vi "Set trigger.vi"(8 "error in (no error)":errorcluster, 11 "StageSPIM in":refnum<class "StageSPIM.lvclass">) -> (0 "error out":errorcluster, 3 "StageSPIM out":refnum<class "StageSPIM.lvclass">)   [LabVIEW 2012, in "StageSPIM.lvclass"]
uses:
  StageSPIM.lvclass
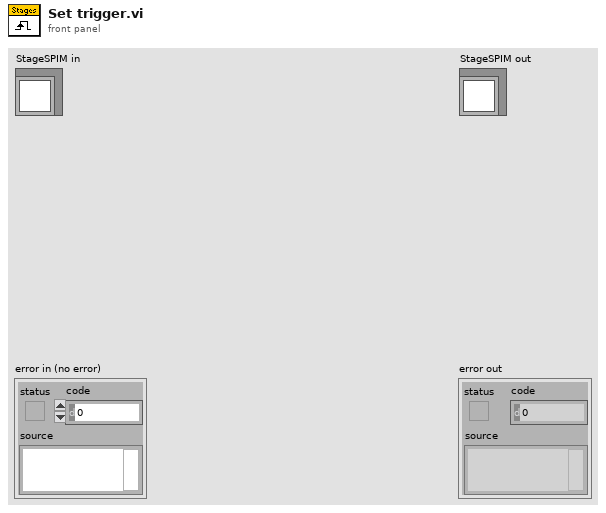
[diagram p1: front panel]
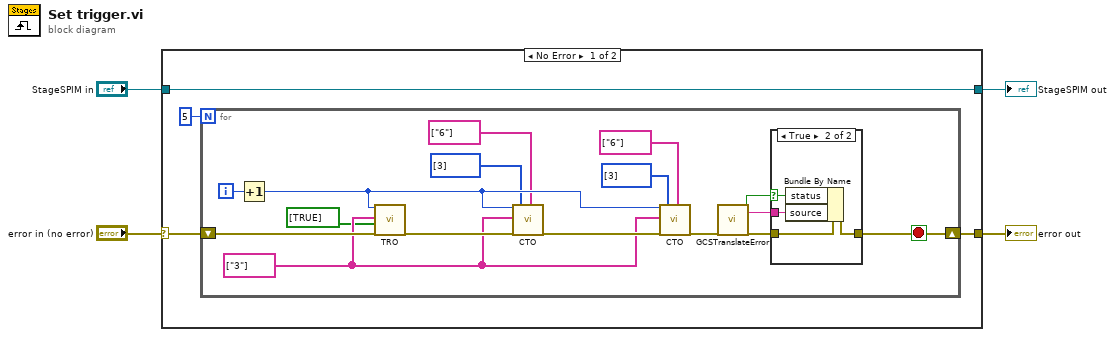
[diagram p0: block diagram]
diagram:
  n1 = case shown="No Error" "error in (no error)" {
    selector: "error in (no error)" -> [w6 w31]
    tunnel: [w5 w31] -> w3
    tunnel: [w8 w30] -> w1
    tunnel: "StageSPIM in" -> [w8 w30]
    frame No Error {
      n2 = for {
        N: 5 -> [_]
        shift-right: [w17] -> w5
        shift-left: w6 -> [w15]
        i -> [w24]
        stop <- w17 stop-if-true
        w13 = string[] ["3"] ("TriggerOut to set")
        n3 = Increment(x=w24) -> (x+1=w12:i32)
        n4 = call "TRO.vi"("System no."=w12, "TriggerOut to command"=w13, "Trigger status"=bool[] [TRUE], "error in"=w15) -> ("error out"=w14:errorcluster)  [unwired: 15 in]
        n5 = call "CTO.vi"("System no."=w12, "TriggerOut to set"=w13, "error in"=w14, "CTO parameter ID"=i32[] [3], "Parameter value"=string[] ["6"]) -> ("error out"=w16:errorcluster)  [unwired: 13 in, 1 out]
        n6 = call "CTO.vi"("System no."=w12, "TriggerOut to set"=w13, "error in"=w16, "CTO parameter ID"=i32[] [3], "Parameter value"=string[] ["6"]) -> ("error out"=w18:errorcluster)  [unwired: 13 in, 1 out]
        n7 = call "GCSTranslateError.vi"("error in"=w18) -> ("GCS Error?"=w20:bool, "Error Description"=w19:string, "error out"=w21:errorcluster)  [unwired: 16 in]
        n8 = case shown="True" w20 {
          selector: w20 -> [_ w27]
          tunnel: w21 -> [w25 w29]
          tunnel: [w25 w28] -> w17
          tunnel: w19 -> [_ w26]
          frame False {
          }
          frame True {
            n9 = Bundle By Name(cluster=w29, "status"=w27, "source"=w26) -> (w28:errorcluster)
          }
        }
      }
    }
    frame Error {
    }
  }
  "error out" <- w3
  "StageSPIM out" <- w1
